vi "Create Manifest File.vi"() -> ()   [LabVIEW 2010]
uses:
  <vilib>/robotics/Simulator/Engine/ctl/Material.ctl
  <vilib>/Utility/miscctls.llb/LV3DPointTypeDef.ctl
  <vilib>/robotics/Simulator/3D-Physics/Plane/3D_Physics_Plane.lvclass
  <vilib>/robotics/Simulator/Engine/ODESimulator_Engine.lvclass
  <vilib>/robotics/Simulator/Robot Classes/Base/ODESimulator_Base_Robot.lvclass
  <vilib>/robotics/Simulator/3D-Physics/Base/3D_Physics_Base.lvclass
  <vilib>/robotics/Simulator/Interface/Simulator Configuration/New Simulation Instance.vi
  <vilib>/robotics/Simulator/Interface/Simulator Configuration/New Environment.vi
  <vilib>/robotics/Simulator/Interface/Simulator Configuration/New Starter Kit 1.0.vi
  <vilib>/robotics/Simulator/NI_Robotics_Simulator.lvlib
panel:
  out "error out":errorcluster
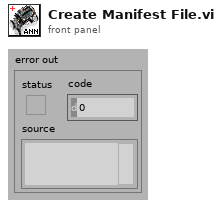
[diagram p1: front panel]
types:
  T1 = typedef "LV3DPointTypeDef.ctl" = cluster{"X":sgl, "Y":sgl, "Z":sgl}
  T2 = typedef "NI_Robotics_Simulator.lvlib/Material.ctl" = enum16{"Smooth", "Copper", "Glass", "Leather", "Rubber", "Steel", "Iron", "Wood", "Stone", "Plastic", "Nylon"}
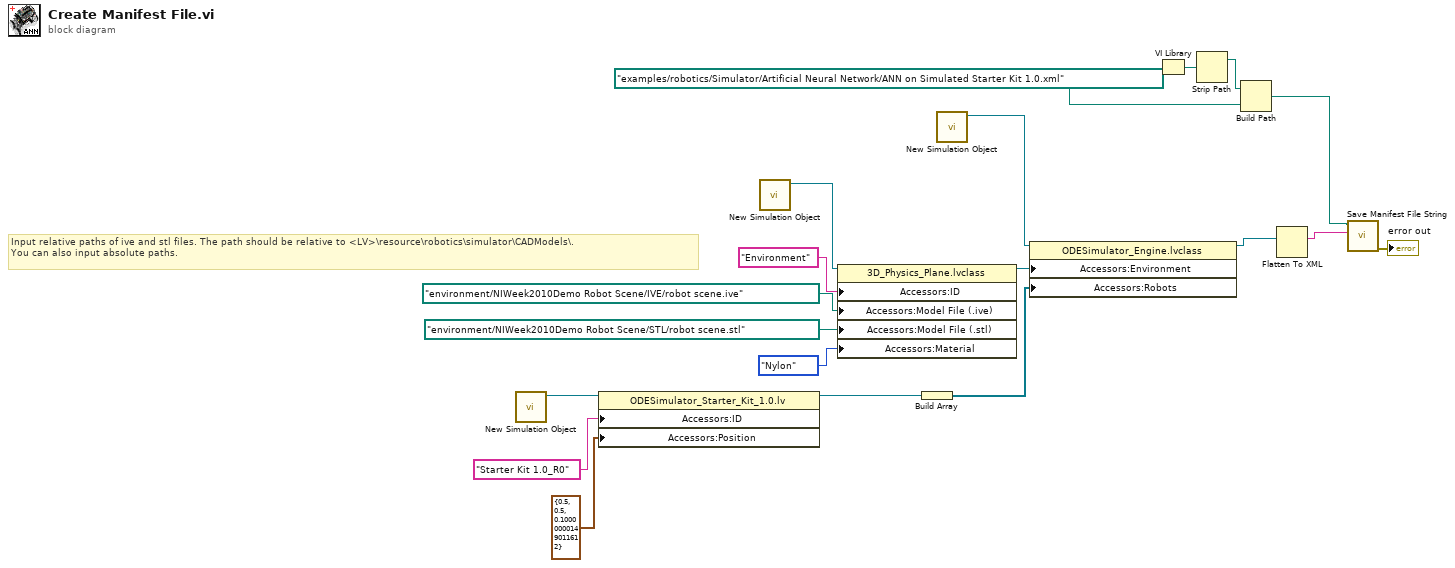
[diagram p0: block diagram]
diagram:
  # "Input relative paths of ive and stl files. The path should be relative to <LV>\\resource\\robotics\\simulator\\CADModels\\.\nYou can also input absolute paths."
  n1 = call-poly <vilib>:"New Simulation Object.vi"() -> ("starter kit 1.0"=w14:refnum<class "ODESimulator_Starter_Kit_1.0.lvclass">)  [unwired: 10 in, 1 out]
  n2 = property class="ODESimulator_Starter_Kit_1.0.lv"(reference=w14, "Accessors:ID"="Starter Kit 1.0_R0" ("ID"), "Accessors:Position"=T1 {"X"=0.5, "Y"=0.5, "Z"=0.1} ("3D Point")) -> (reference out=w9:refnum<class "ODESimulator_Starter_Kit_1.0.lvclass">)  [unwired: 1 in, 1 out]
  n3 = call-poly <vilib>:"New Simulation Object.vi"() -> ("environment"=w19:refnum<class "3D_Physics_Plane.lvclass">)  [unwired: 10 in, 1 out]
  n4 = property class="3D_Physics_Plane.lvclass"(reference=w19, "Accessors:ID"="Environment" ("ID"), "Accessors:Model File (.ive)"=path "environment/NIWeek2010Demo Robot Scene/IVE/robot scene.ive" ("Visual Model File"), "Accessors:Model File (.stl)"=path "environment/NIWeek2010Demo Robot Scene/STL/robot scene.stl" ("Physics Model File"), "Accessors:Material"=Material."Nylon" ("Material")) -> (reference out=w10:refnum<class "3D_Physics_Plane.lvclass">)  [unwired: 1 in, 1 out]
  n5 = Build Array(w9) -> (w8:refnum<class "ODESimulator_Starter_Kit_1.0.lvclass">[])
  n6 = call-poly <vilib>:"New Simulation Object.vi"() -> ("simulation instance"=w11:refnum<class "ODESimulator_Engine.lvclass">)  [unwired: 10 in, 1 out]
  n7 = property class="ODESimulator_Engine.lvclass"(reference=w11, "Accessors:Environment"=w10, "Accessors:Robots"=w8) -> (reference out=w4:refnum<class "ODESimulator_Engine.lvclass">)  [unwired: 1 in, 1 out]
  n8 = VI Library() -> (path=w5:path)
  n9 = Strip Path(path=w5) -> (stripped path=w6:path)  [unwired: 1 out]
  n10 = Build Path(base path=w6, name or relative path=path "examples/robotics/Simulator/Artificial Neural Network/ANN on Simulated Starter Kit 1.0.xml" ("path")) -> (appended path=w3:path)
  n11 = Flatten To XML(anything=w4) -> (xml string=w1:string)
  n12 = call <vilib>:"Save Manifest File String.vi"("manifest file string"=w1, "manifest file path"=w3) -> ("error out"=→"error out":errorcluster)  [unwired: 9 in]
